vi "tlc_Timing Module.vi"(4 "Cue States":T1[][](array[typedef]), 6 "Update Rate":u32, 7 "Command":T4, 8 "error in (no error)":errorcluster, 9 "Cue Input":T2 {"Channels"."Intensity" min=0.0 max=100.0 step=1.0 format="%#.0f"}, 10 "Play Structure Names":T5) -> (0 "error out":errorcluster, 1 "Cue Output":T2 {"Channels"."Intensity" min=0.0 max=100.0 step=1.0 format="%#.0f"}, 2 "Update Rate Out":u32)   [LabVIEW 2018]
uses:
  Controls/Play Structure Names.ctl
  tlc_Timing Command Control.ctl
  Controls/tlc_Cue_Information.ctl
  Controls/channel.ctl
  Controls/Cue State.ctl
  <vilib>/Platform/TimedLoop/XDataNode/timing_clust.ctl
  <vilib>/Platform/TimedLoop/XDataNode/nitl_modes.ctl
  <vilib>/Platform/TimedLoop/XDataNode/wakeup.ctl
  <vilib>/Platform/TimedLoop/scheduler/LVUserAPI/_suppVIs/Create_1kHz_TSource.vi
  <vilib>/Platform/TimedLoop/XDataNode/XDataNode.xnode
  <vilib>/Platform/TimedLoop/XDataNode/XDNodeRunTimeDep.lvlib
panel:
  # "Input"
  # "Internal Data"
  # "Output"
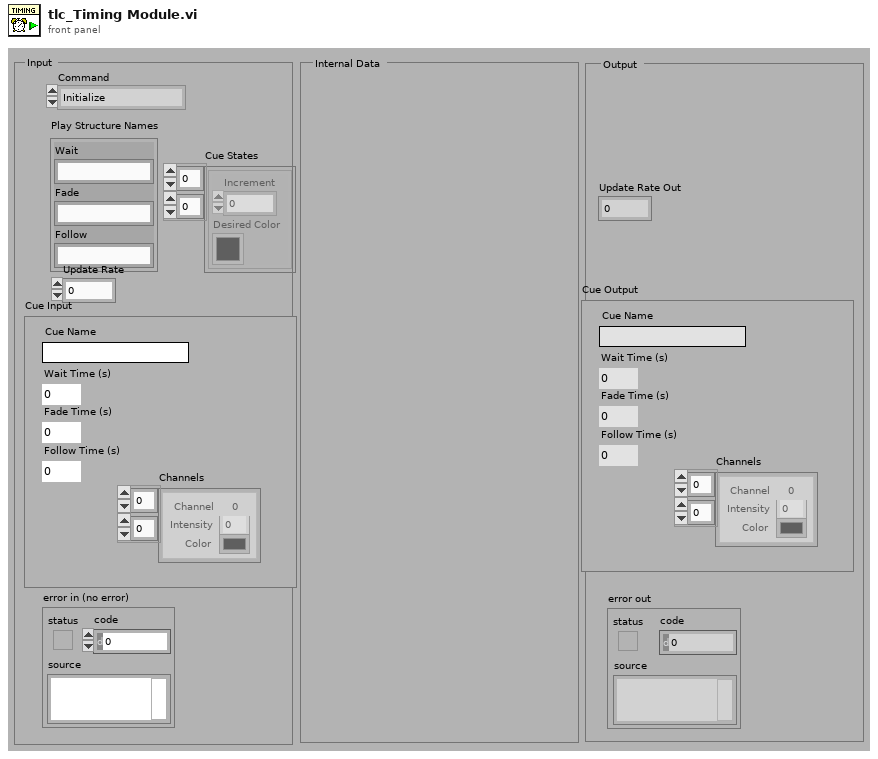
[diagram p1: front panel]
types:
  T1 = typedef "Cue State.ctl" = cluster{"Increment":dbl, "Desired Color":u32}
  T2 = typedef "tlc_Cue_Information.ctl" = cluster{"Cue Name":string, "Wait Time (s)":u32, "Fade Time (s)":u32, "Follow Time (s)":u32, "Channels":T3[][]}
  T3 = typedef "channel.ctl" = cluster{"Intensity":dbl, " Color":u32, "Channel":i32}
  T4 = typedef "tlc_Timing Command Control.ctl" = enum16{"Initialize", "Get Information", "Create", "Wait", "Fade", "Follow", "Shutdown"}
  T5 = typedef "Play Structure Names.ctl" = cluster{"Wait":string, "Fade":string, "Follow":string}
  T6 = typedef "XDNodeRunTimeDep.lvlib/timing_clust.ctl" = cluster{"Expected End [f-1]":u64, "Actual End [f-1]":u64, "Finished Late? [f-1]":bool, "Expected End [i-1]":u64, "Actual End [i-1]":u64, "Finished Late? [i-1]":bool, "Expected Start [i]":u64, "Actual Start [i]":u64, "Expected Start [f]":u64, "Actual Start [f]":u64, "Source Name":string, "Structure Name":string, "Period":i64, "Deadline":i64, "Offset":i64, "Start":i64, "Priority":i32, "Timeout":i32, "Mode":T7, "Wakeup Reason":T8, "Error":errorcluster, "Source Type":string, "Secondary Source Type":string, "Global End Time":u64, "Global Start Time":u64, "Frame Duration":u64, "Iteration Duration":u64, "Assigned CPU":i32, "I/O Scan Engine Mode":u32}
  T7 = typedef "XDNodeRunTimeDep.lvlib/nitl_modes.ctl" = enum32{"No Change", "Process missed periods, maintain original phase", "Discard missed periods, maintain original phase", "Process missed periods, ignore original phase", "Discard missed periods, ignore original phase"}
  T8 = typedef "XDNodeRunTimeDep.lvlib/wakeup.ctl" = enum32{"Normal", "Aborted", "Asynchronous wakeup", "Timing source error", "Timed loop error", "Timeout"}
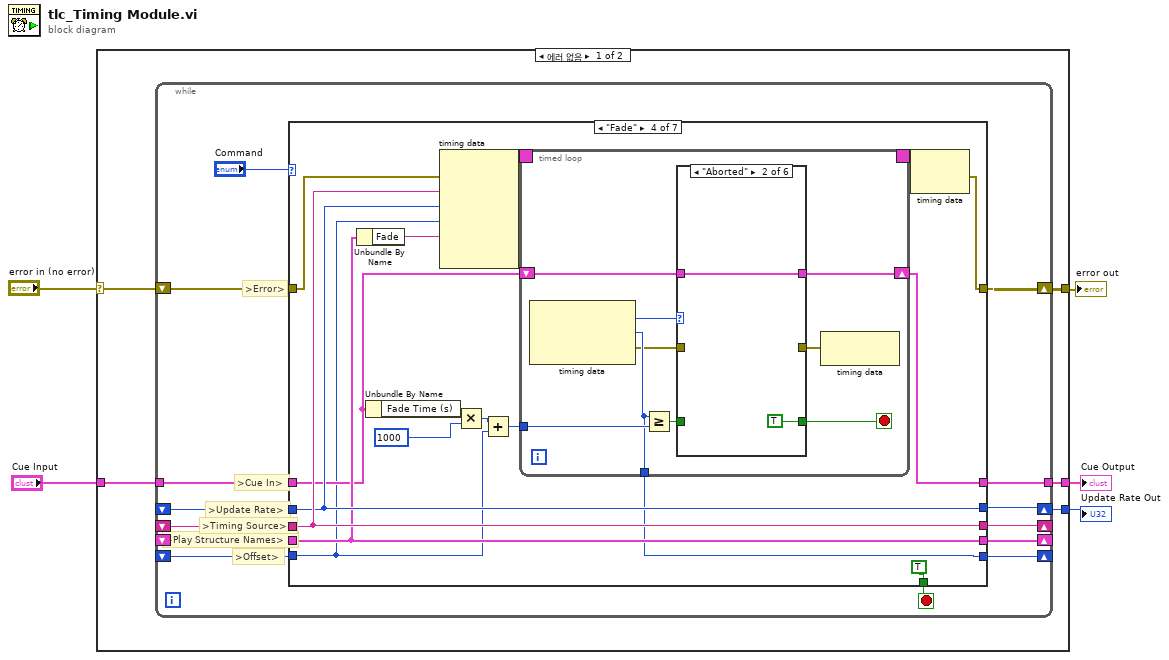
[diagram p0: block diagram]
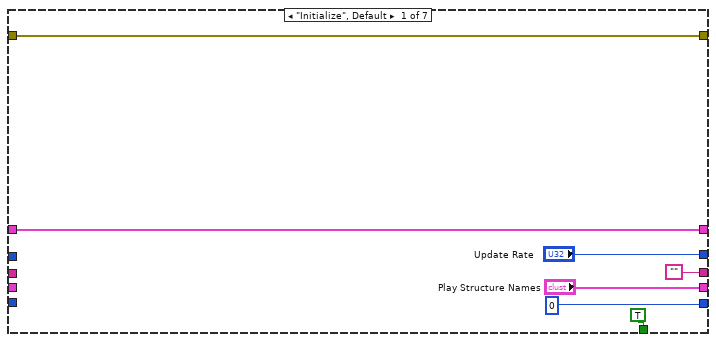
[diagram p2: hidden frame]
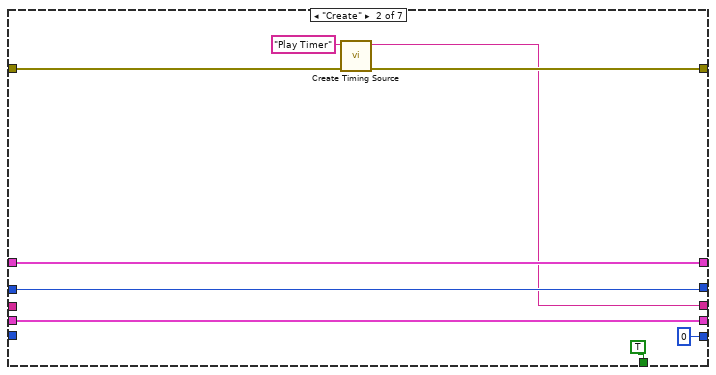
[diagram p3: hidden frame]
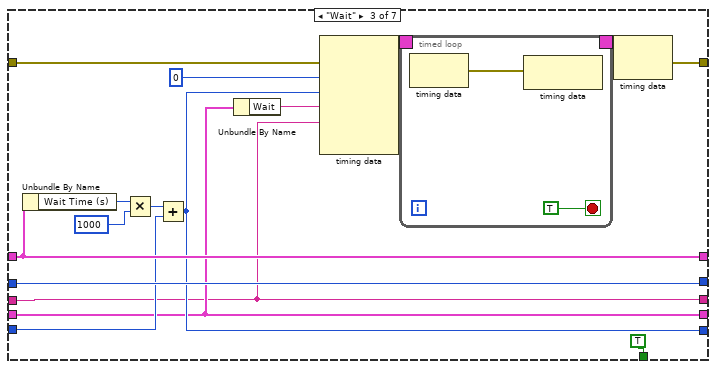
[diagram p4: hidden frame]
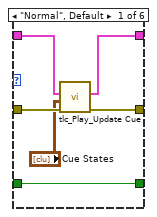
[diagram p5: hidden frame]
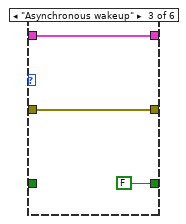
[diagram p6: hidden frame]
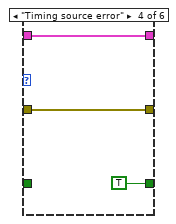
[diagram p7: hidden frame]
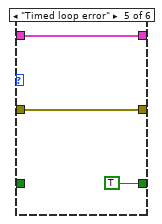
[diagram p8: hidden frame]
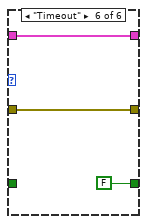
[diagram p9: hidden frame]
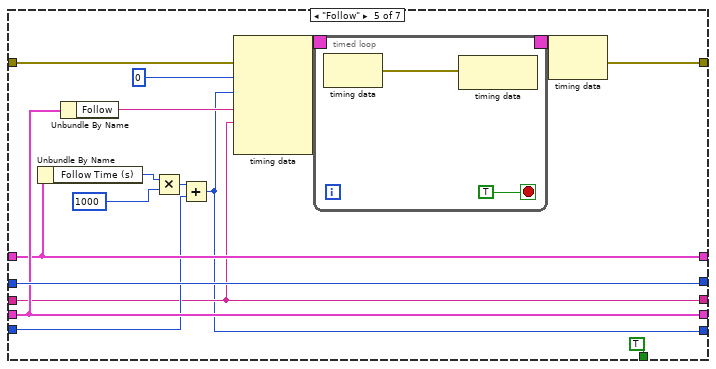
[diagram p10: hidden frame]
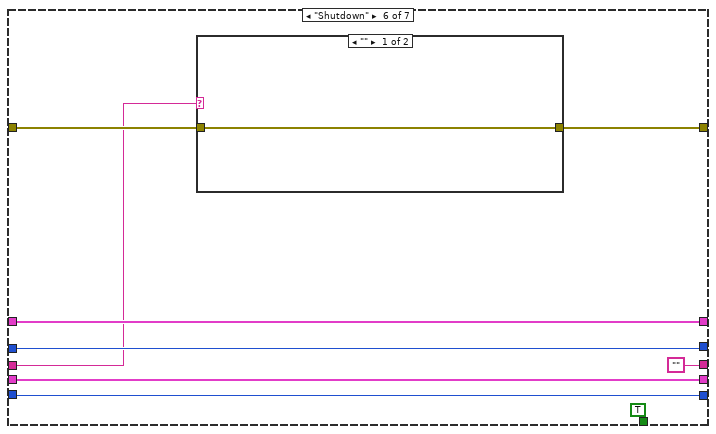
[diagram p11: hidden frame]
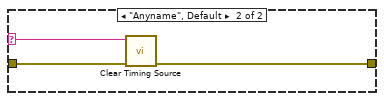
[diagram p12: hidden frame]
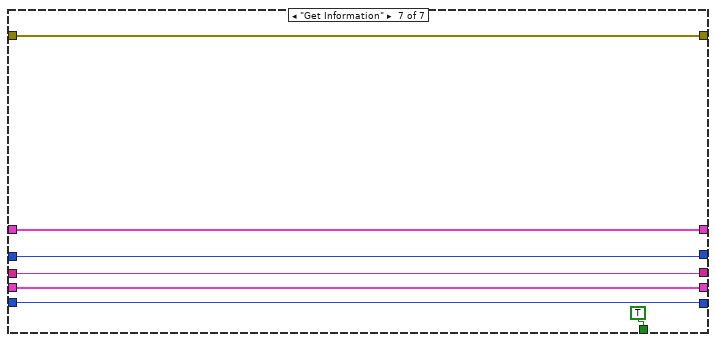
[diagram p13: hidden frame]
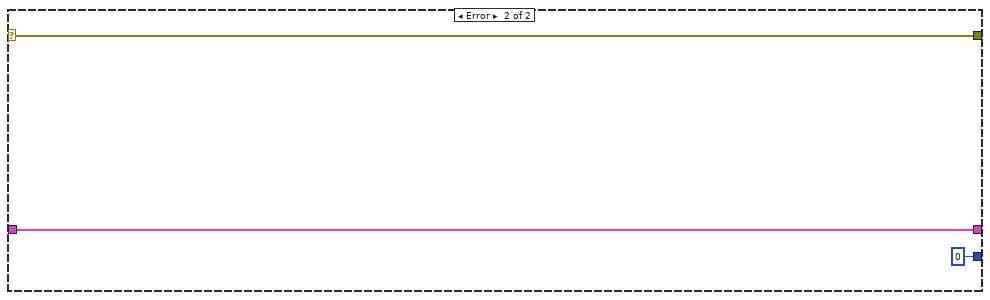
[diagram p14: hidden frame]
diagram:
  n1 = case shown="에러 없음" "error in (no error)" {
    selector: "error in (no error)" -> [w10 w189]
    tunnel: [w9 w189] -> w4
    tunnel: "Cue Input" -> [w8 w188]
    tunnel: [w7 w188] -> w2
    tunnel: [w6 u32 0 ("Update Rate")] -> w1
    frame No Error {
      n2 = while {
        shift-right: [w23] -> w9
        shift-left: w10 -> [w24]
        shift-right: [w22] -> _
        shift-left: _ -> [w21]
        shift-right: [w20] -> _
        shift-left: _ -> [w19]
        shift-right: [w18] -> w6
        shift-left: _ -> [w17]
        shift-right: [w16] -> _
        shift-left: _ -> [w15]
        tunnel: w8 -> [w12]
        tunnel: [w11] -> w7
        stop <- w14 stop-if-true
        # ">Error>"
        # ">Cue In>"
        # ">Offset>"
        # ">Update Rate>"
        # ">Play Structure Names>"
        # ">Timing Source>"
        n3 = case shown="\"Fade\"" "Command" {
          tunnel: w24 -> [w25 w35 w52 w86 w145 w171 w181]
          tunnel: [w25 w34 w51 w73 w146 w169 w181] -> w23
          tunnel: ["" ("name (out)") w32 w41 w85 w136 "" w184] -> w22
          tunnel: w21 -> [_ _ w41 w85 w136 w170 w184]
          tunnel: ["Play Structure Names" w39 w43 w83 w143 w173 w185] -> w20
          tunnel: w19 -> [_ w39 w43 w83 w143 w173 w185]
          tunnel: ["Update Rate" w40 w56 w84 w150 w174 w183] -> w18
          tunnel: w17 -> [_ w40 w56 w84 w150 w174 w183]
          tunnel: [u32 0 u32 0 w44 w75 w135 w168 w186] -> w16
          tunnel: w15 -> [_ _ w45 w77 w137 w168 w186]
          tunnel: [TRUE TRUE TRUE TRUE TRUE TRUE TRUE] -> w14
          tunnel: [w26 w37 w49 w74 w141 w172 w182] -> w11
          tunnel: w12 -> [w26 w37 w49 w81 w141 w172 w182]
          frame "Initialize", Default {
          }
          frame "Create" {
            n4 = call-poly <vilib>:"Create Timing Source.vi"("error in (no error)"=w35, "name (in)"="Play Timer") -> ("error out"=w34:errorcluster, "name (out)"=w32:string)  [unwired: 8 in]
          }
          frame "Wait" {
            n5 = Unbundle By Name(w49) -> ("Wait Time (s)"=w48:u32)
            n6 = Multiply(x=w48, y=u32 1000) -> (x*y=w46:u32)
            n7 = Add(x=w46, y=w45) -> (x+y=w44:i64)
            n8 = Unbundle By Name(w43) -> ("Wait"=w42:string)
            n9 = node-c288(w52, i64 0 ("Period"), w44, w42, w41) -> (w54:T6)  [unwired: 1 in]
            n10 = timed-loop {
              timing: w54 -> [_]
              timing-out: [_] -> w53
              stop <- TRUE stop-if-true
              n11 = node-c288() -> (w57:errorcluster)  [unwired: 1 in]
              n12 = node-c288(w57) -> ()  [unwired: 1 out]
            }
            n13 = node-c288(w53) -> (w51:errorcluster)
          }
          frame "Fade" {
            n14 = Unbundle By Name(w83) -> ("Fade"=w82:string)
            n15 = Unbundle By Name(w81) -> ("Fade Time (s)"=w80:u32)
            n16 = node-c288(w86, w85, w84, w77, w82) -> (w88:T6)  [unwired: 1 in]
            n17 = Multiply(x=w80, y=u32 1000) -> (x*y=w78:u32)
            n18 = Add(x=w78, y=w77) -> (x+y=w76:i64)
            n19 = timed-loop {
              timing: w88 -> [_]
              timing-out: [_] -> w87
              shift-right: [w90] -> w74
              shift-left: w81 -> [w91]
              tunnel: w76 -> [w97]
              tunnel: [w96] -> w75
              stop <- w94 stop-if-true
              n20 = node-c288() -> (w98:T8, w96:i64, w93:errorcluster)  [unwired: 1 in]
              n21 = Greater Or Equal?(x=w96, y=w97) -> (x >= y?=w95:bool)
              n22 = case shown="\"Aborted\"" w98 {
                tunnel: w95 -> [w104 _ _ _ _ _]
                tunnel: [w104 TRUE FALSE TRUE TRUE FALSE] -> w94
                tunnel: w93 -> [w101 _ w109 w111 w114 w117]
                tunnel: [w100 _ w109 w111 w114 w117] -> w92
                tunnel: w91 -> [w103 w105 w108 w110 w115 w118]
                tunnel: [w102 w105 w108 w110 w115 w118] -> w90
                frame "Normal", Default {
                  n23 = call "tlc_Play_Update Cue.vi"("error in"=w101, "Cue States"="Cue States", "Cue Input"=w103) -> ("error out"=w100:errorcluster, "Cue Output"=w102:T2)  [unwired: 7 in]
                }
                frame "Aborted" {
                }
                frame "Asynchronous wakeup" {
                }
                frame "Timing source error" {
                }
                frame "Timed loop error" {
                }
                frame "Timeout" {
                }
              }
              n24 = node-c288(w92) -> ()  [unwired: 1 out]
            }
            n25 = node-c288(w87) -> (w73:errorcluster)
          }
          frame "Follow" {
            n26 = Unbundle By Name(w141) -> ("Follow Time (s)"=w140:u32)
            n27 = Unbundle By Name(w143) -> ("Follow"=w142:string)
            n28 = Multiply(x=w140, y=u32 1000) -> (x*y=w138:u32)
            n29 = Add(x=w138, y=w137) -> (x+y=w135:i64)
            n30 = node-c288(w145, i64 0 ("Period"), w135, w142, w136) -> (w148:T6)  [unwired: 1 in]
            n31 = timed-loop {
              timing: w148 -> [_]
              timing-out: [_] -> w147
              stop <- TRUE stop-if-true
              n32 = node-c288() -> (w151:errorcluster)  [unwired: 1 in]
              n33 = node-c288(w151) -> ()  [unwired: 1 out]
            }
            n34 = node-c288(w147) -> (w146:errorcluster)
          }
          frame "Shutdown" {
            n35 = case shown="\"\"" w170 {
              selector: w170 -> [_ w179]
              tunnel: w171 -> [w176 w178]
              tunnel: [w176 w177] -> w169
              frame "" {
              }
              frame "Anyname", Default {
                n36 = call <vilib>:"Clear Timing Source.vi"("error in (no error)"=w178, "name"=w179) -> ("error out"=w177:errorcluster)  [unwired: 8 in, 1 out]
              }
            }
          }
          frame "Get Information" {
          }
        }
      }
    }
    frame Error {
    }
  }
  "error out" <- w4
  "Cue Output" <- w2
  "Update Rate Out" <- w1
